vi "Win Filepath-use or create v3.vi"(5 "Dir Path":path, 6 "error in":errorcluster, 7 "File Name":string, 8 "Subdir":string, 9 "Win Directory Type":T1=1 items=["User Home"=0, "User Desktop"=1, "User Documents"=2, "User Application Data"=3, "User Preferences"=4, "User Temporary"=5, "Public Documents"=6, "Public Application Data"=7, "Public Preferences"=8, "Public Cache"=13, "System Core Libraries"=9, "System Installed Libraries"=10, "Application Files"=11, "Boot Volume Root"=12]) -> (0 "error out":errorcluster, 3 "Filepath":path)   [LabVIEW 2020]
uses:
  System Directory Type.ctl
panel:
  # "If Dir Path isnot empty and valid, simply use that and Filename  to create Filepath. Otherwise if Subdir is provided, either create or use existing Subdir in WIndows directory.  If no Subdir provided then use Win Dir"
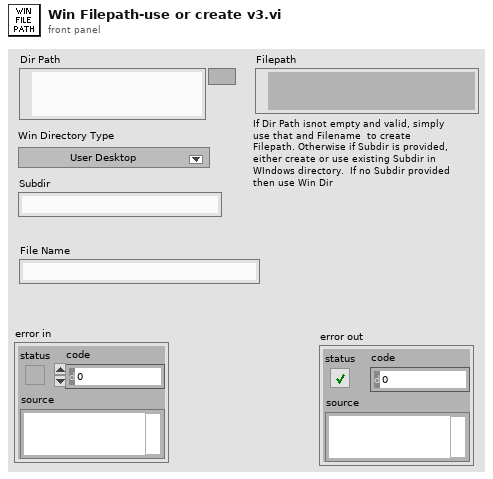
[diagram p1: front panel]
types:
  T1 = typedef "System Directory Type.ctl" = i32
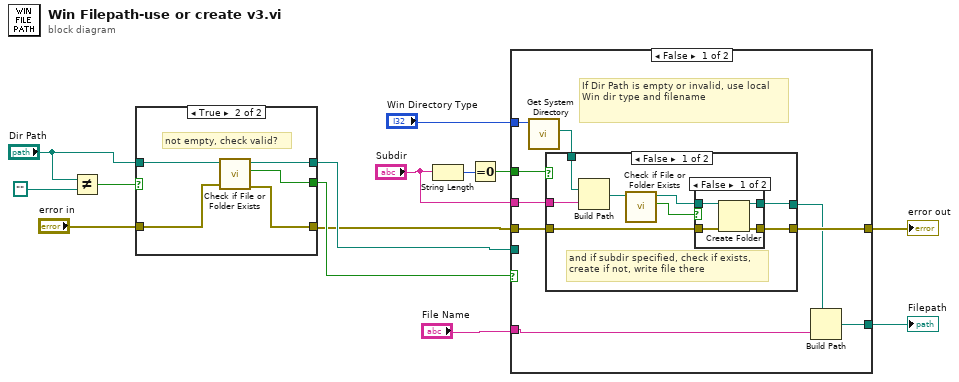
[diagram p0: block diagram]
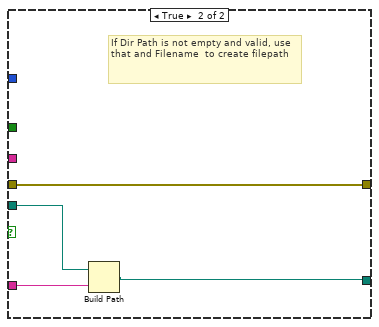
[diagram p5: hidden frame]
diagram:
  n1 = Not Equal?(x="Dir Path", y=path "") -> (x != y?=w4:bool)
  n2 = case shown="True" w4 {
    selector: w4 -> [w17 _]
    tunnel: [w16 w22] -> w7
    tunnel: [w17 w21] -> w6
    tunnel: "Dir Path" -> [w16 w20]
    tunnel: "error in" -> [w15 w19]
    tunnel: [w15 w18] -> w1
    frame False {
      # "empty"
    }
    frame True {
      # "not empty, check valid?"
      n3 = call "Check if File or Folder Exists.vi"("error in (no error)"=w19, "path"=w20) -> ("error out"=w18:errorcluster, "file or folder exists?"=w21:bool, "dup path"=w22:path)  [unwired: 7 in]
    }
  }
  n4 = String Length(string="Subdir") -> (length=w12:i32)
  n5 = Equal To 0?(x=w12) -> (x = 0?=w11:bool)
  n6 = case shown="False" w6 {
    tunnel: [w31 w48] -> w8
    tunnel: "File Name" -> [w23 w50]
    tunnel: w7 -> [_ w49]
    tunnel: "Win Directory Type" -> [w30 _]
    tunnel: w11 -> [w29 _]
    tunnel: "Subdir" -> [w28 _]
    tunnel: w1 -> [w26 w51]
    tunnel: [w25 w51] -> w9
    frame False {
      # "If Dir Path is empty or invalid, use local Win dir type and filename"
      n7 = call "Get System Directory.vi"("system directory type"=w30) -> ("system directory"=w27:path)  [unwired: 10 in]
      n8 = case shown="False" w29 {
        tunnel: w28 -> [w39 _]
        tunnel: w27 -> [w38 w47]
        tunnel: w26 -> [w34 w46]
        tunnel: [w33 w46] -> w25
        tunnel: [w32 w47] -> w24
        frame False {
          # "and if subdir specified, check if exists,\ncreate if not, write file there"
          n9 = Build Path(base path=w38, name or relative path=w39) -> (appended path=w37:path)
          n10 = call "Check if File or Folder Exists.vi"("path"=w37) -> ("file or folder exists?"=w36:bool, "dup path"=w35:path)  [unwired: 8 in, 1 out]
          n11 = case shown="False" w36 {
            tunnel: w35 -> [w43 w44]
            tunnel: w34 -> [w42 w45]
            tunnel: [w41 w45] -> w33
            tunnel: [w40 w44] -> w32
            frame False {
              n12 = Create Folder(path (use dialog)=w43, error in=w42) -> (created path=w40:path, error out=w41:errorcluster)  [unwired: 1 in, 1 out]
            }
            frame True {
            }
          }
        }
        frame True {
          # "and Subdir string is empty, write file to\nspecified windows directory"
        }
      }
      n13 = Build Path(base path=w24, name or relative path=w23) -> (appended path=w31:path)
    }
    frame True {
      # "If Dir Path is not empty and valid, use that and Filename  to create filepath"
      n14 = Build Path(base path=w49, name or relative path=w50) -> (appended path=w48:path)
    }
  }
  "error out" <- w9
  "Filepath" <- w8
